vi "funguje_cteni_slow_fast.vi"() -> ()   [LabVIEW 2022 SP3]
uses:
  controls/State_control.ctl
  controls/Data.ctl
  <vilib>/Utility/sysdir.llb/System Directory Type.ctl
panel:
  out "Doba mereni [ms]":i16
  in  "Pocet vz":i8
  in  "vzorky/s":enum16{"Slow", "2F2F"}(ring)
  out "amp":string[](array[string])
  out "volt":string[](array[string])
  out "single amp":string
  out "single volt":string
  out "IDN commnad 4":string
  in  "GPD-3303S":refnum<visa-resource-name>
  in  "Stop":bool
  in  "Store data":bool
  in  "Reset array":bool
  in  "Start meas":bool
  out "IDN commnad":string
  in  "Agilent 34401A":refnum<visa-resource-name>
  in  "Agilent 34450A":refnum<visa-resource-name>
  out "IDN commnad 3":string
  out "State":T1=enum."SaveData"
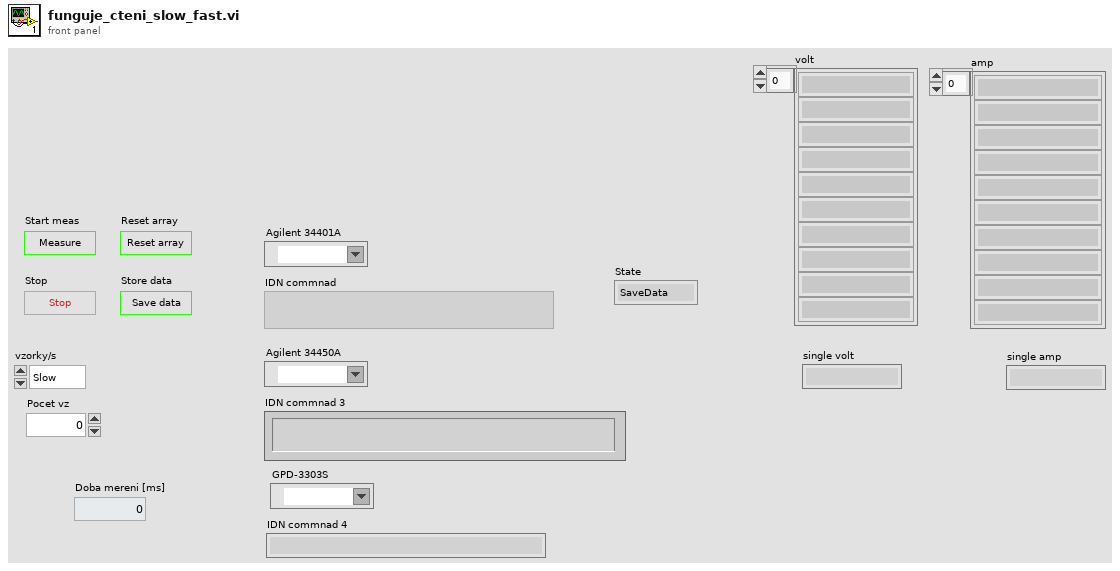
[diagram p1: front panel]
types:
  T1 = typedef "State_control.ctl" = enum16{"Init", "Waiting", "Measure", "SaveData", "Finish"}
  T2 = typedef "Data.ctl" = cluster{"Meas Samples":i32, "Samples/s":i32, "Averaging":i32, "TC_Voltage":dbl[], "TC_Temperature":dbl[], "PT_Resistance":dbl[], "PT_Temperature":dbl[], "TC_Temperature_compen":dbl[], "Date":string[], "Time":string[]}
  T3 = cluster{"Agilent 34401A":refnum<visa-resource-name>, "Agilent 34450A":refnum<visa-resource-name>}
  T4 = typedef "System Directory Type.ctl" = i32
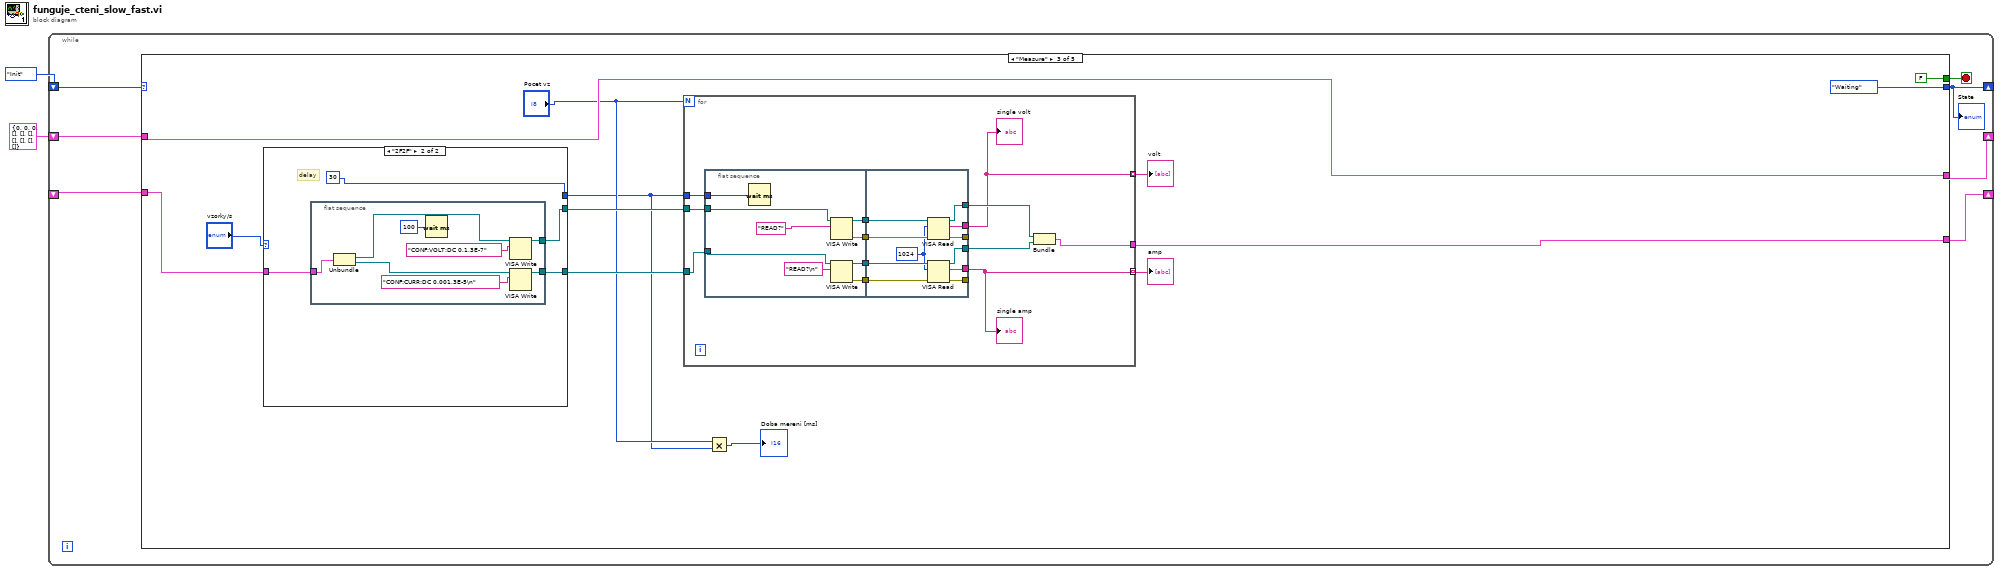
[diagram p0: block diagram]
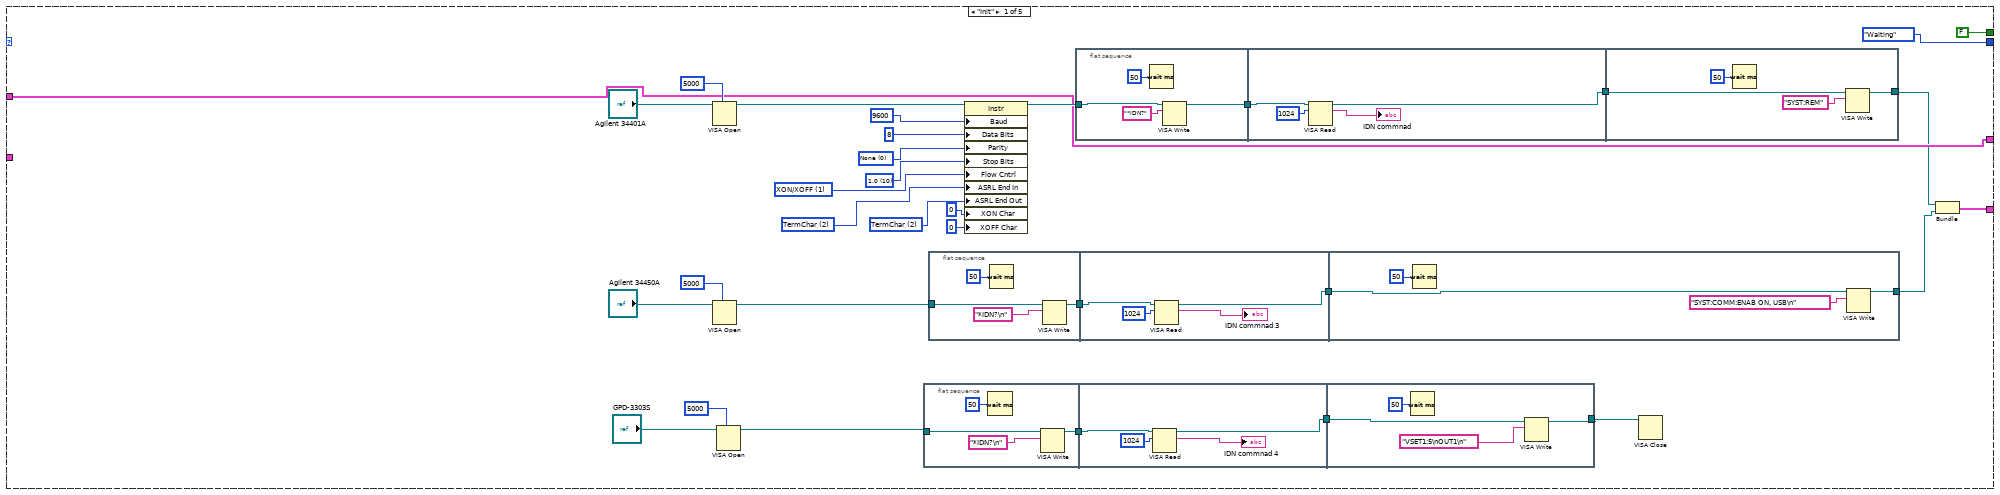
[diagram p2: hidden frame]
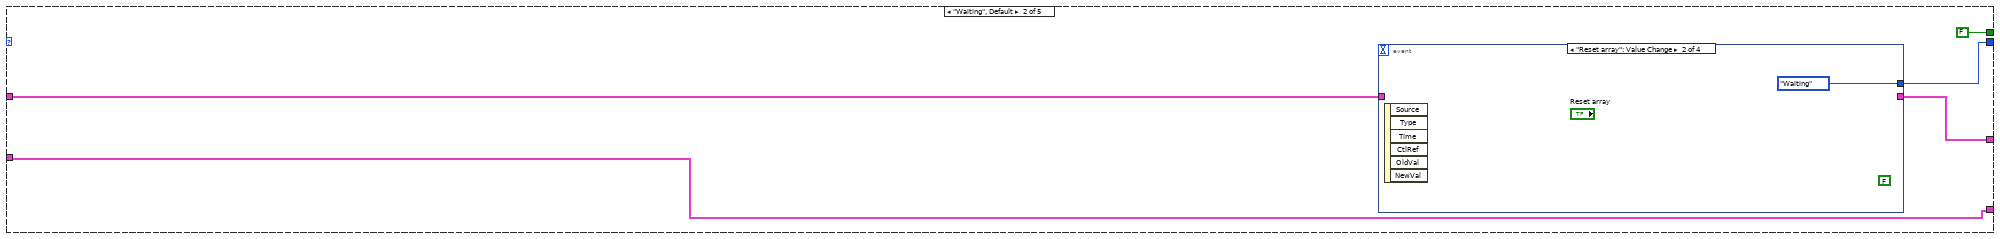
[diagram p3: hidden frame]
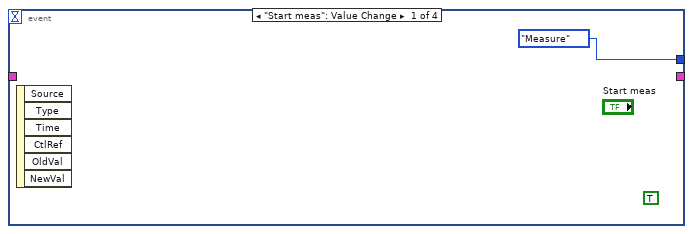
[diagram p4: hidden frame]
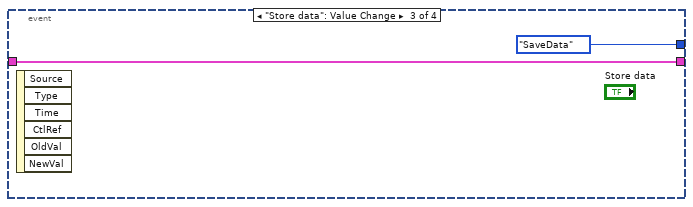
[diagram p5: hidden frame]
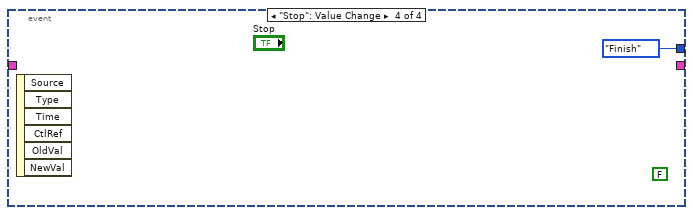
[diagram p6: hidden frame]
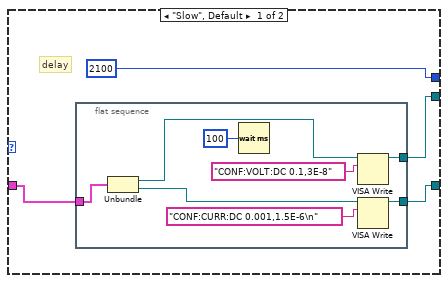
[diagram p7: hidden frame]
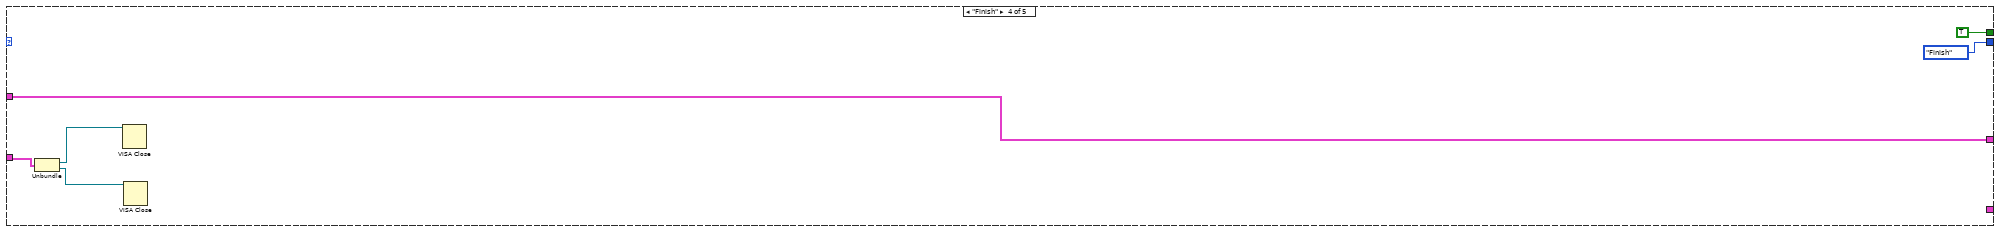
[diagram p8: hidden frame]
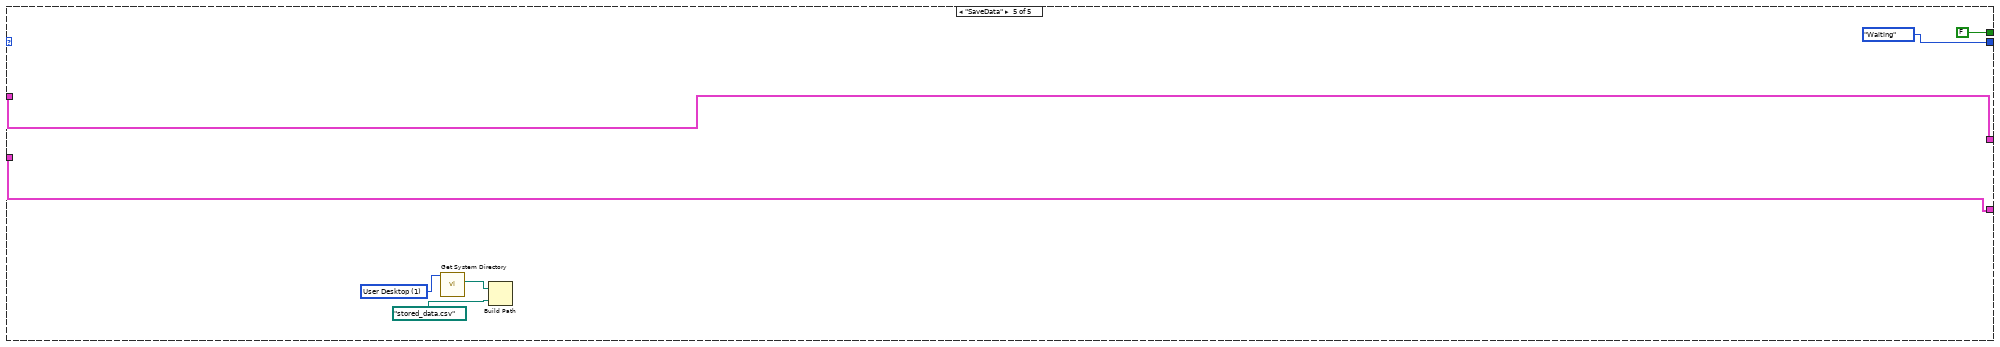
[diagram p9: hidden frame]
diagram:
  n1 = while {
    shift-right: [w3] -> _
    shift-left: State_control."Init" ("State") -> [w9]
    shift-right: [w6] -> _
    shift-left: T2 {"Meas Samples"=0, "Samples/s"=0, "Averaging"=0, "TC_Voltage"=[], "TC_Temperature"=[], "PT_Resistance"=[], "PT_Temperature"=[], "TC_Temperature_compen"=[], "Date"=[], "Time"=[]} ("Data") -> [w7]
    shift-right: [w5] -> _
    shift-left: _ -> [w4]
    stop <- w8 stop-if-true
    n2 = case shown="\"Measure\"" w9 {
      tunnel: [State_control."Waiting" ("State 2") w79 State_control."Waiting" ("State 2") State_control."Finish" ("State 2") State_control."Waiting" ("State 2")] -> w3
      tunnel: [FALSE FALSE FALSE TRUE FALSE] -> w8
      tunnel: w7 -> [w26 w78 w94 w160 w163]
      tunnel: [w26 w81 w94 w160 w163] -> w6
      tunnel: [w11 w80 w95 _ w167] -> w5
      tunnel: w4 -> [_ w80 w98 w159 w167]
      frame "Init" {
        w31 = u16 2 items=["None", "Last Bit", "TermChar", "Break"] ("Serial Settings:End Mode for Writes")
        w32 = u16 2 items=["None", "Last Bit", "TermChar"] ("Serial Settings:End Mode for Reads")
        w33 = u16 1 items=["None", "XON/XOFF", "RTS/CTS", "XON/XOFF & RTS/CTS", "DTR/DSR", "XON/XOFF & DTR/DSR"] ("Serial Settings:Flow Control")
        w34 = u16 10 items=["1.0"=10, "1.5"=15, "2.0"=20] ("Serial Settings:Stop Bits")
        w35 = u16 0 items=["None", "Odd", "Even", "Mark", "Space"] ("Serial Settings:Parity")
        n3 = VISA Open(timeout (0)=u32 5000 ("VISA Open timeout (0)"), VISA resource name="Agilent 34401A") -> (VISA resource name=w38:refnum<visa-resource-name>)  [unwired: 3 in, 1 out]
        n4 = VISA Open(timeout (0)=u32 5000 ("VISA Open timeout (0)"), VISA resource name="Agilent 34450A") -> (VISA resource name=w19:refnum<visa-resource-name>)  [unwired: 3 in, 1 out]
        n5 = VISA Open(timeout (0)=u32 5000 ("VISA Open timeout (0)"), VISA resource name="GPD-3303S") -> (VISA resource name=w14:refnum<visa-resource-name>)  [unwired: 3 in, 1 out]
        n6 = flat-sequence {
          tunnel: [w44] -> w16
          tunnel: w14 -> [w42]
          tunnel: w16 -> [w48]
          tunnel: [w47] -> w15
          tunnel: [w50] -> w10
          tunnel: w15 -> [w51]
          frame #0 {
            n7 = Wait (ms)(milliseconds to wait=u32 50) -> ()  [unwired: 1 out]
            n8 = VISA Write(VISA resource name=w42, write buffer="*IDN?\n") -> (VISA resource name out=w44:refnum<visa-resource-name>)  [unwired: 1 in, 2 out]
          }
          frame #1 {
            n9 = VISA Read(VISA resource name=w48, byte count=u32 1024) -> (VISA resource name out=w47:refnum<visa-resource-name>, read buffer=→"IDN commnad 4":string)  [unwired: 1 in, 2 out]
          }
          frame #2 {
            n10 = Wait (ms)(milliseconds to wait=u32 50) -> ()  [unwired: 1 out]
            n11 = VISA Write(VISA resource name=w51, write buffer="VSET1:5\nOUT1\n") -> (VISA resource name out=w50:refnum<visa-resource-name>)  [unwired: 1 in, 2 out]
          }
        }
        n12 = flat-sequence {
          tunnel: [w56] -> w23
          tunnel: w19 -> [w54]
          tunnel: w23 -> [w60]
          tunnel: [w59] -> w22
          tunnel: [w62] -> w12
          tunnel: w22 -> [w63]
          frame #0 {
            n13 = Wait (ms)(milliseconds to wait=u32 50) -> ()  [unwired: 1 out]
            n14 = VISA Write(VISA resource name=w54, write buffer="*IDN?\n") -> (VISA resource name out=w56:refnum<visa-resource-name>)  [unwired: 1 in, 2 out]
          }
          frame #1 {
            n15 = VISA Read(VISA resource name=w60, byte count=u32 1024) -> (VISA resource name out=w59:refnum<visa-resource-name>, read buffer=→"IDN commnad 3":string)  [unwired: 1 in, 2 out]
          }
          frame #2 {
            n16 = Wait (ms)(milliseconds to wait=u32 50) -> ()  [unwired: 1 out]
            n17 = VISA Write(VISA resource name=w63, write buffer="SYST:COMM:ENAB ON, USB\n") -> (VISA resource name out=w62:refnum<visa-resource-name>)  [unwired: 1 in, 2 out]
          }
        }
        n18 = property class="Instr"(reference=w38, "Baud"=u32 9600 ("Serial Settings:Baud Rate"), "Data Bits"=u16 8 ("Serial Settings:Data Bits"), "Parity"=w35, "Stop Bits"=w34, "Flow Cntrl"=w33, "ASRL End In"=w32, "ASRL End Out"=w31, "XON Char"=u8 0 ("Serial Settings:Flow Control XON Character"), "XOFF Char"=u8 0 ("Serial Settings:Flow Control XOFF Character")) -> (reference out=w27:refnum<visa-resource-name>)  [unwired: 1 in, 1 out]
        n19 = flat-sequence {
          tunnel: w27 -> [w69]
          tunnel: [w67] -> w28
          tunnel: w28 -> [w72]
          tunnel: [w71] -> w25
          tunnel: [w75] -> w13
          tunnel: w25 -> [w76]
          frame #0 {
            n20 = Wait (ms)(milliseconds to wait=u32 50) -> ()  [unwired: 1 out]
            n21 = VISA Write(VISA resource name=w69, write buffer="*IDN?") -> (VISA resource name out=w67:refnum<visa-resource-name>)  [unwired: 1 in, 2 out]
          }
          frame #1 {
            n22 = VISA Read(VISA resource name=w72, byte count=u32 1024) -> (VISA resource name out=w71:refnum<visa-resource-name>, read buffer=→"IDN commnad":string)  [unwired: 1 in, 2 out]
          }
          frame #2 {
            n23 = Wait (ms)(milliseconds to wait=u32 50) -> ()  [unwired: 1 out]
            n24 = VISA Write(VISA resource name=w76, write buffer="SYST:REM") -> (VISA resource name out=w75:refnum<visa-resource-name>)  [unwired: 1 in, 2 out]
          }
        }
        n25 = VISA Close(VISA resource name=w10) -> ()  [unwired: 1 in, 1 out]
        n26 = Bundle("Agilent 34401A"=w13, "Agilent 34450A"=w12) -> (w11:T3)  [unwired: 1 in]
      }
      frame "Waiting", Default {
        n27 = event shown="[1] \"Reset array\": Value Change" {
          selector: _ -> [_ _ _ _]
          dyn-events: _ -> [_ _ _ _]
          timeout: _ -> [_ _ _ _]
          tunnel: [State_control."Measure" ("State 2") State_control."Waiting" ("State 2") State_control."SaveData" ("State 2") State_control."Finish" ("State 2")] -> w79
          tunnel: w78 -> [_ _ w85 _]
          tunnel: [_ _ w85 _] -> w81
          event "Start meas": Value Change {
            (unwired) TRUE
            n28 = event-data() -> ()  [unwired: 1 in, 6 out]
          }
          event "Reset array": Value Change {
            (unwired) FALSE
            n29 = event-data() -> ()  [unwired: 1 in, 6 out]
          }
          event "Store data": Value Change {
            n30 = event-data() -> ()  [unwired: 1 in, 6 out]
          }
          event "Stop": Value Change {
            (unwired) FALSE
            n31 = event-data() -> ()  [unwired: 1 in, 6 out]
          }
        }
      }
      frame "Measure" {
        n32 = case shown="\"2F2F\"" "vzorky/s" {
          tunnel: w98 -> [w104 w116]
          tunnel: [w101 w115] -> w97
          tunnel: [w102 w114] -> w96
          tunnel: [u32 2100 ("milliseconds to wait") u32 30 ("milliseconds to wait")] -> w89
          frame "Slow", Default {
            # "delay"
            n33 = flat-sequence {
              tunnel: [w110] -> w102
              tunnel: w104 -> [w107]
              tunnel: [w109] -> w101
              frame #0 {
                n34 = Unbundle(w107) -> ("Agilent 34401A"=w106:refnum<visa-resource-name>, "Agilent 34450A"=w105:refnum<visa-resource-name>)
                n35 = Wait (ms)(milliseconds to wait=u32 100) -> ()  [unwired: 1 out]
                n36 = VISA Write(VISA resource name=w106, write buffer="CONF:VOLT:DC 0.1,3E-8") -> (VISA resource name out=w110:refnum<visa-resource-name>)  [unwired: 1 in, 2 out]
                n37 = VISA Write(VISA resource name=w105, write buffer="CONF:CURR:DC 0.001,1.5E-6\n") -> (VISA resource name out=w109:refnum<visa-resource-name>)  [unwired: 1 in, 2 out]
              }
            }
          }
          frame "2F2F" {
            # "delay"
            n38 = flat-sequence {
              tunnel: [w122] -> w114
              tunnel: w116 -> [w119]
              tunnel: [w121] -> w115
              frame #0 {
                n39 = Unbundle(w119) -> ("Agilent 34401A"=w118:refnum<visa-resource-name>, "Agilent 34450A"=w117:refnum<visa-resource-name>)
                n40 = Wait (ms)(milliseconds to wait=u32 100) -> ()  [unwired: 1 out]
                n41 = VISA Write(VISA resource name=w118, write buffer="CONF:VOLT:DC 0.1,3E-7") -> (VISA resource name out=w122:refnum<visa-resource-name>)  [unwired: 1 in, 2 out]
                n42 = VISA Write(VISA resource name=w117, write buffer="CONF:CURR:DC 0.001,3E-5\n") -> (VISA resource name out=w121:refnum<visa-resource-name>)  [unwired: 1 in, 2 out]
              }
            }
          }
        }
        n43 = for {
          N: "Pocet vz" -> [_]
          tunnel: w97 -> [w132]
          tunnel: w96 -> [w131]
          tunnel: [w128] -> w95
          tunnel: [w127] -> w93 mode=indexing
          tunnel: [w126] -> w92 mode=indexing
          tunnel: w89 -> [w125]
          n44 = flat-sequence {
            tunnel: [w145] -> w136
            tunnel: w131 -> [w144]
            tunnel: [w143] -> w135
            tunnel: w132 -> [w142]
            tunnel: [w141] -> w134
            tunnel: [w140] -> w133
            tunnel: w125 -> [w137]
            tunnel: w136 -> [w155]
            tunnel: [w156] -> w130
            tunnel: [w154] -> w127
            tunnel: [w153] -> _
            tunnel: w135 -> [w152]
            tunnel: w134 -> [w151]
            tunnel: w133 -> [w150]
            tunnel: [w149] -> w129
            tunnel: [w148] -> w126
            tunnel: [w147] -> _
            frame #0 {
              n45 = Wait (ms)(milliseconds to wait=w137) -> ()  [unwired: 1 out]
              n46 = VISA Write(VISA resource name=w144, write buffer="READ?") -> (VISA resource name out=w145:refnum<visa-resource-name>, error out=w143:errorcluster)  [unwired: 1 in, 1 out]
              n47 = VISA Write(VISA resource name=w142, write buffer="READ?\n") -> (VISA resource name out=w140:refnum<visa-resource-name>, error out=w141:errorcluster)  [unwired: 1 in, 1 out]
            }
            frame #1 {
              w146 = u32 1024 ("byte count")
              n48 = VISA Read(VISA resource name=w155, byte count=w146, error in (no error)=w152) -> (VISA resource name out=w156:refnum<visa-resource-name>, read buffer=w154:string, error out=w153:errorcluster)  [unwired: 1 out]
              n49 = VISA Read(VISA resource name=w150, byte count=w146, error in (no error)=w151) -> (VISA resource name out=w149:refnum<visa-resource-name>, read buffer=w148:string, error out=w147:errorcluster)  [unwired: 1 out]
            }
          }
          n50 = Bundle("Agilent 34401A"=w130, "Agilent 34450A"=w129) -> (w128:T3)  [unwired: 1 in]
          "single volt" <- w127
          "single amp" <- w126
        }
        "volt" <- w93
        "amp" <- w92
        n51 = Multiply(x="Pocet vz", y=w89) -> (x*y=→"Doba mereni [ms]":u32)
      }
      frame "Finish" {
        n52 = Unbundle(w159) -> ("Agilent 34401A"=w158:refnum<visa-resource-name>, "Agilent 34450A"=w157:refnum<visa-resource-name>)
        n53 = VISA Close(VISA resource name=w158) -> ()  [unwired: 1 in, 1 out]
        n54 = VISA Close(VISA resource name=w157) -> ()  [unwired: 1 in, 1 out]
      }
      frame "SaveData" {
        w166 = T4 1 items=["User Home"=0, "User Desktop"=1, "User Documents"=2, "User Application Data"=3, "User Preferences"=4, "User Temporary"=5, "Public Documents"=6, "Public Application Data"=7, "Public Preferences"=8, "Public Cache"=13, "System Core Libraries"=9, "System Installed Libraries"=10, "Application Files"=11, "Boot Volume Root"=12] ("system directory type")
        n55 = call <vilib>:"Get System Directory.vi"("system directory type"=w166) -> ("system directory"=w164:path)  [unwired: 10 in]
        n56 = Build Path(base path=w164, name or relative path=path "stored_data.csv") -> ()  [unwired: 1 out]
      }
    }
    "State" <- w3
  }
